vi "AH_EvalSTB.vi"(8 "error in (no error)":errorcluster, 9 "Status Byte":T1 items=["ONR"=1, "CME"=2, "URQ"=4, "PON"=8, "RDY"=16, "EXE"=32, "RQS"=64, "MAV"=128], 10 "Data Cluster In":T2 {"GUI Data Cluster"."SBR" format="%08b"}, 11 "Config Cluster In":T4={"General"={"Config.ini"=path "", "Default Logging Path"=path ""}, "Hardware"={"Measure Rate (1/s)"=0, "HP DMM VISA"="", "LS 335 VISA"="", "HP DM"={"Range"=enum."Autorange", "Autozero"=FALSE, "Display"=enum."3 1/2 Digit", "Blank LCD"=FALSE}}, "Operation"={"Operation Mode"=enum."Logging", "Status"="", "NewLog?"=FALSE, "OvenWarn"=FALSE}}) -> (0 "error out":errorcluster, 1 "Result":bool, 2 "Data Cluster Out":T2 {"GUI Data Cluster"."SBR" format="%08b"}, 3 "Configuration Cluster Out":T4={"General"={"Config.ini"=path "", "Default Logging Path"=path ""}, "Hardware"={"Measure Rate (1/s)"=0, "HP DMM VISA"="", "LS 335 VISA"="", "HP DM"={"Range"=enum."Autorange", "Autozero"=FALSE, "Display"=enum."3 1/2 Digit", "Blank LCD"=FALSE}}, "Operation"={"Operation Mode"=enum."Idle-Off", "Status"="", "NewLog?"=FALSE, "OvenWarn"=FALSE}}, 4 "Total Result":bool[](array[boolean]))   [LabVIEW 2021]
uses:
  Mode_Enum.ctl
  Config_Cluster.ctl
  Measurement_Cluster.ctl
  Data_Cluster.ctl
  Status_Byte.ctl
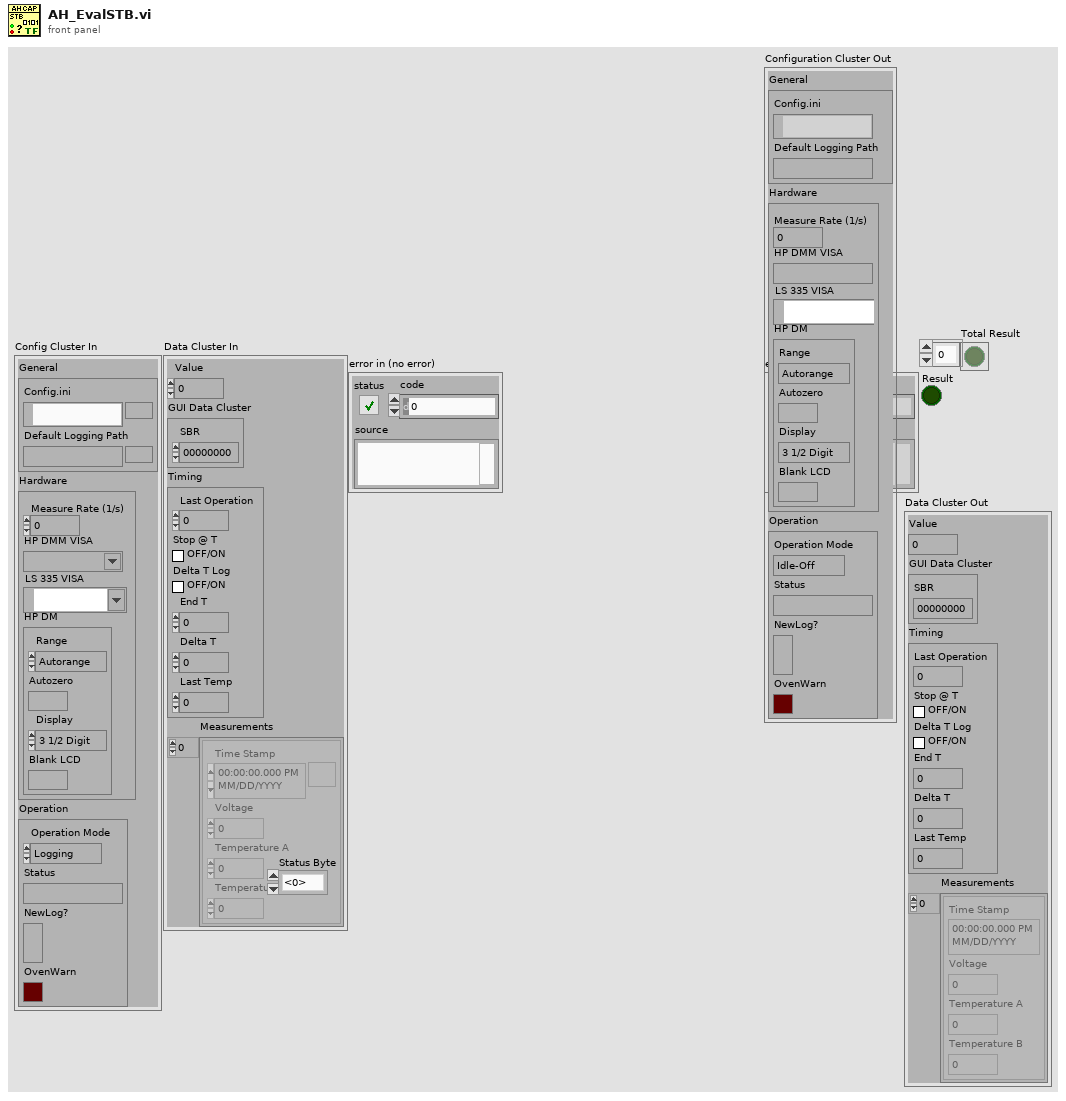
[diagram p1: front panel]
types:
  T1 = typedef "Status_Byte.ctl" = u16
  T2 = typedef "Data_Cluster.ctl" = cluster{"Value":dbl, "GUI Data Cluster":cluster{"SBR":u16}, "Timing":cluster{"Last Operation":dbl, "Stop @ T":bool, "Delta T Log":bool, "End T":dbl, "Delta T":dbl, "Last Temp":dbl}, "Measurements":T3[]}
  T3 = typedef "Measurement_Cluster.ctl" = cluster{"Time Stamp":timestamp, "Voltage":dbl, "Temperature A":dbl, "Temperature B":dbl}
  T4 = typedef "Config_Cluster.ctl" = cluster{"General":cluster{"Config.ini":path, "Default Logging Path":path}, "Hardware":cluster{"Measure Rate (1/s)":i32, "HP DMM VISA":refnum<visa-resource-name>, "LS 335 VISA":refnum<visa-resource-name>, "HP DM":cluster{"Range":enum16{"Autorange", "30mV", "300mV", "3V", "30V"}, "Autozero":bool, "Display":enum16{"3 1/2 Digit", "4 1/2 Digit", "5 1/2 Digit"}, "Blank LCD":bool}}, "Operation":cluster{"Operation Mode":T5, "Status":string, "NewLog?":bool, "OvenWarn":bool}}
  T5 = typedef "Mode_Enum.ctl" = enum16{"OvenNRDY", "Logging", "Idle-Off", "Idle"}
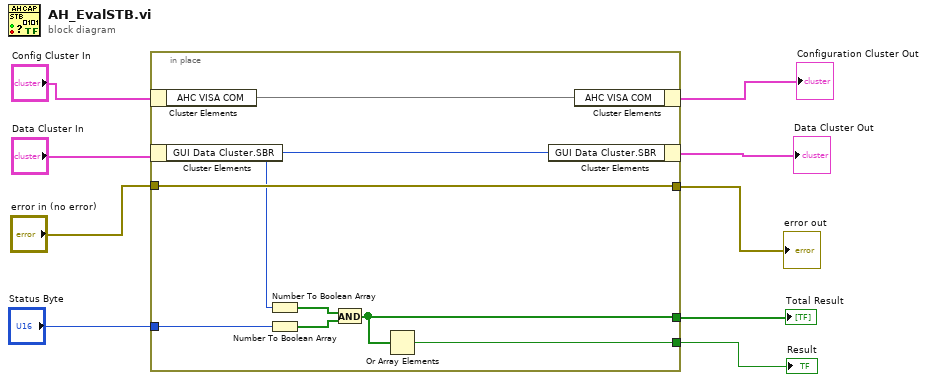
[diagram p0: block diagram]
diagram:
  n1 = in-place {
    in-place-border: "error in (no error)" -> [w16]
    in-place-border: [w16] -> w6
    in-place-border: "Status Byte" -> [w15]
    in-place-border: [w11] -> w2
    in-place-border: [w10] -> w1
    n2 = in-place-cluster #1("Config Cluster In") -> ("AHC VISA COM"=w17)
    n3 = in-place-cluster #2("Data Cluster In") -> ("GUI Data Cluster.SBR"=w14:u16)
    n4 = Number To Boolean Array(number=w14) -> (Boolean array=w13:bool[])
    n5 = Number To Boolean Array(number=w15) -> (Boolean array=w12:bool[])
    n6 = And(x=w13, y=w12) -> (x .and. y?=w11:bool[])
    n7 = Or Array Elements(Boolean array=w11) -> (logical OR=w10:bool)
    n8 = in-place-cluster #2("GUI Data Cluster.SBR"=w14) -> (→"Data Cluster Out":T2)
    n9 = in-place-cluster #1("AHC VISA COM"=w17) -> (→"Configuration Cluster Out":T4)
  }
  "error out" <- w6
  "Total Result" <- w2
  "Result" <- w1
